vi "HandleTabTEST.vi"(8 "error in (no error)":errorcluster, 11 "S4GUI in":refnum<class "S4GUI.lvclass">) -> (0 "error out":errorcluster, 3 "S4GUI out":refnum<class "S4GUI.lvclass">)   [LabVIEW 2018, in "S4GUI.lvclass"]
uses:
  S4GUI.lvclass
  S4GUI.lvclass/S4GUI.ctl
  Instrument/Instrument.lvclass/Instrument.ctl
  Device/Optics/Optics.lvclass/Optics.ctl
  Device/Optics/Opt_Selector/Opt_Selector.lvclass
  C:/Users/devstaff/sparc4/s4gui/Versao ZeroMQ REQ-REP/SPARC4_GUI -v1.0.9 - novo comportamento aba TEST/Device/Optics/Optics.lvclass
  Acquisition/Acquisition.lvclass
  Instrument/Instrument.lvclass
  Channel/Channel.lvclass
  Interface/Interface.lvclass
  Device/Optics/Optics.lvclass
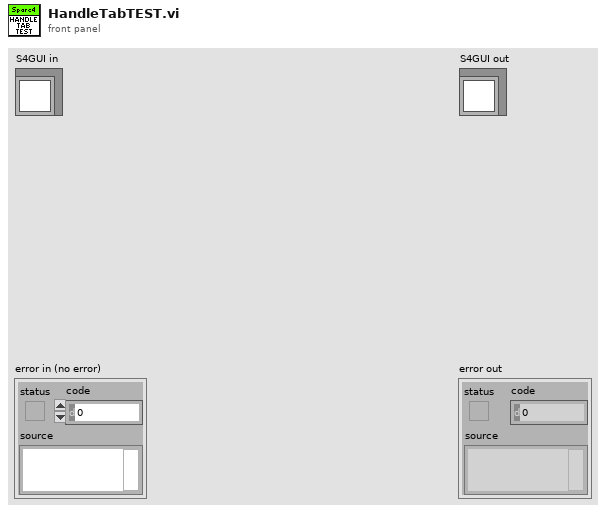
[diagram p1: front panel]
types:
  T1 = enum32{"OBJECT", "TEST", "DFLAT", "SFLAT", "DARK", "ZERO", "FOCUS"}
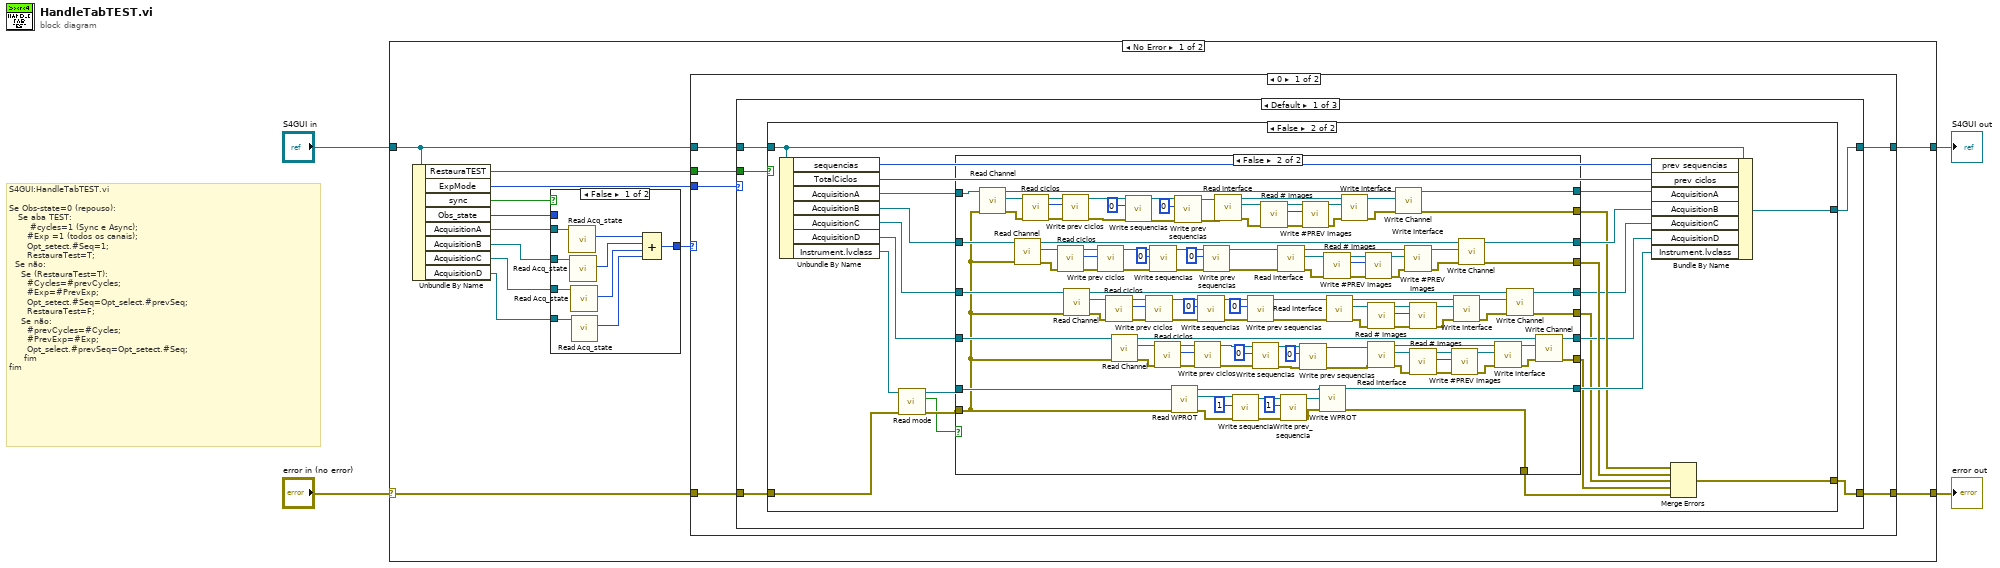
[diagram p0: block diagram]
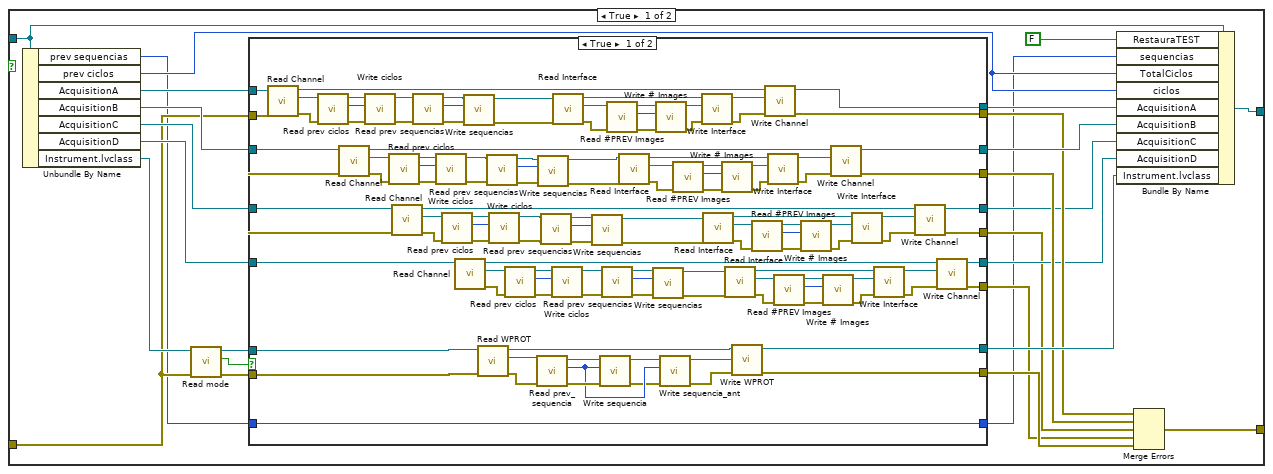
[diagram p3: hidden frame]
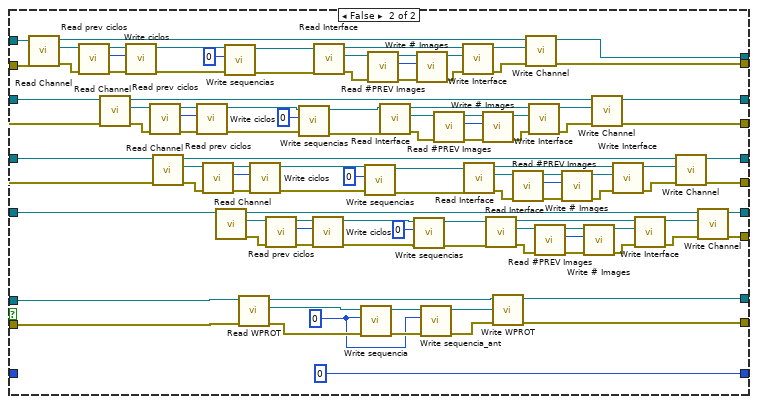
[diagram p4: hidden frame]
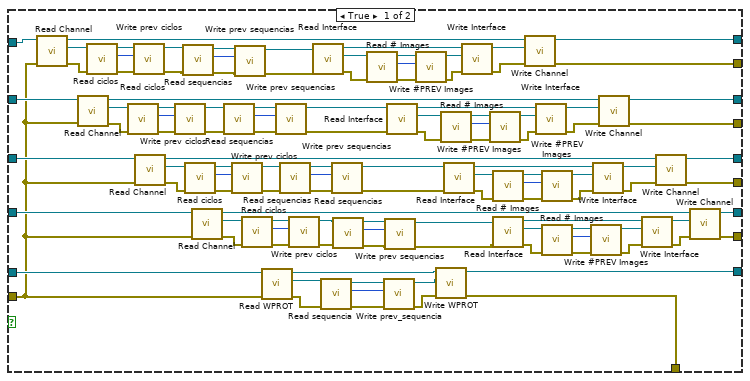
[diagram p5: hidden frame]
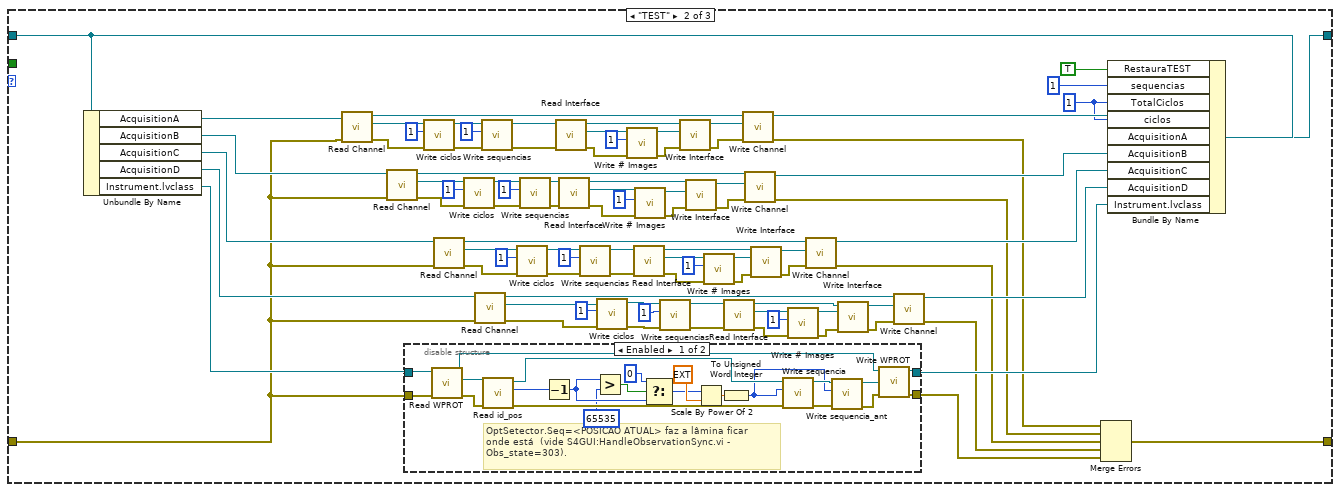
[diagram p6: hidden frame]
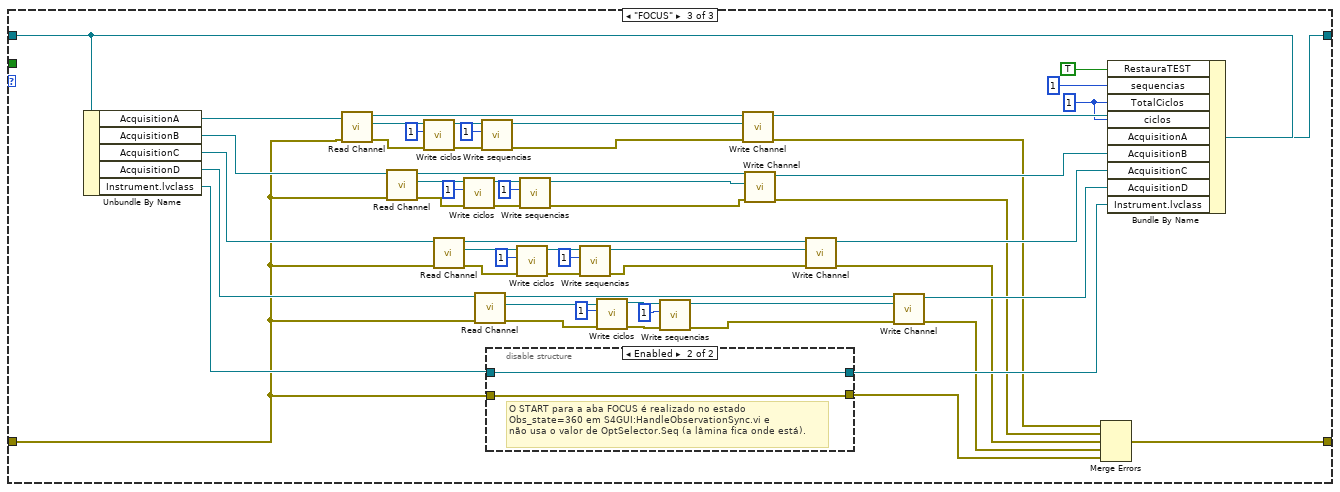
[diagram p8: hidden frame]
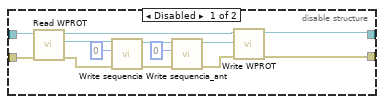
[diagram p9: hidden frame]
diagram:
  # "S4GUI:HandleTabTEST.vi\n\nSe Obs-state=0 (repouso):\n   Se aba TEST: \n       #cycles=1 (Sync e Async);\n      #Exp =1 (todos os canais);\n      Opt_setect.#Seq=1;\n      RestauraTest=T;\n  Se não:\n    Se (RestauraTest=T):\n      #Cycles=#prevCycles;\n      #Exp=#PrevExp;\n      Opt_setect.#Seq=Opt_select.#prevSeq;\n      RestauraTest=F;\n    Se não:\n      #prevCycles=#Cycles;\n      #PrevExp=#Exp;\n      Opt_select.#prevSeq=Opt_setect.#Seq;\n     fim\nfim"
  n1 = case shown="No Error" "error in (no error)" {
    selector: "error in (no error)" -> [w17 w746]
    tunnel: [w14 w746] -> w3
    tunnel: [w15 w745] -> w1
    tunnel: "S4GUI in" -> [w16 w745]
    frame No Error {
      n2 = Unbundle By Name(w16) -> ("RestauraTEST"=w5:bool, "ExpMode"=w7:T1, "sync"=w6:bool, "Obs_state"=w13:u32, "AcquisitionA"=w12:refnum<class "Acquisition.lvclass">, "AcquisitionB"=w11:refnum<class "Acquisition.lvclass">, "AcquisitionC"=w10:refnum<class "Acquisition.lvclass">, "AcquisitionD"=w9:refnum<class "Acquisition.lvclass">)
      n3 = case shown="False" w6 {
        tunnel: w13 -> [_ w27]
        tunnel: w12 -> [w26 _]
        tunnel: w11 -> [w24 _]
        tunnel: w10 -> [w23 _]
        tunnel: w9 -> [w22 _]
        tunnel: [w18 w27] -> w8
        frame False {
          n4 = call-dynamic "Read Acq_state.vi"("Acquisition in"=w26) -> ("Acq_state"=w25:u32)  [unwired: 8 in, 2 out]
          n5 = call-dynamic "Read Acq_state.vi"("Acquisition in"=w24) -> ("Acq_state"=w21:u32)  [unwired: 8 in, 2 out]
          n6 = call-dynamic "Read Acq_state.vi"("Acquisition in"=w23) -> ("Acq_state"=w20:u32)  [unwired: 8 in, 2 out]
          n7 = call-dynamic "Read Acq_state.vi"("Acquisition in"=w22) -> ("Acq_state"=w19:u32)  [unwired: 8 in, 2 out]
          n8 = Compound Arithmetic op=ADD(w25, w21, w20, w19) -> (w18:u32)
        }
        frame True {
        }
      }
      n9 = case shown="0" w8 {
        tunnel: w17 -> [w30 w743]
        tunnel: [w31 w744] -> w15
        tunnel: w16 -> [w32 w744]
        tunnel: [w29 w743] -> w14
        tunnel: w7 -> [w33 _]
        tunnel: w5 -> [w28 _]
        frame 0 {
          n10 = case shown="Default" w33 {
            tunnel: w32 -> [w37 w604 w710]
            tunnel: [w34 w603 w709] -> w31
            tunnel: w30 -> [w36 w590 w700]
            tunnel: [w35 w584 w694] -> w29
            tunnel: w28 -> [w38 _ _]
            frame Default {
              n11 = case shown="False" w38 {
                tunnel: w37 -> [w55 w308]
                tunnel: w36 -> [w45 w298]
                tunnel: [w56 w309] -> w35
                tunnel: [w54 w307] -> w34
                frame True {
                  n12 = Unbundle By Name(w55) -> ("prev sequencias"=w40:u32, "prev ciclos"=w42:u32, "AcquisitionA"=w64:refnum<class "Acquisition.lvclass">, "AcquisitionB"=w61:refnum<class "Acquisition.lvclass">, "AcquisitionC"=w53:refnum<class "Acquisition.lvclass">, "AcquisitionD"=w52:refnum<class "Acquisition.lvclass">, "Instrument.lvclass"=w46:refnum<class "Instrument.lvclass">)
                  n13 = call-dynamic "Read mode.vi"("error in (no error)"=w45, "Instrument in"=w46) -> ("error out"=w43:errorcluster, "mode"=w41:bool, "Instrument out"=w44:refnum<class "Instrument.lvclass">)  [unwired: 7 in]
                  n14 = case shown="True" w41 {
                    tunnel: w64 -> [w184 w294]
                    tunnel: [w178 w288] -> w63
                    tunnel: [w177 w287] -> w62
                    tunnel: w61 -> [w152 w262]
                    tunnel: [w148 w258] -> w60
                    tunnel: [w147 w257] -> w59
                    tunnel: [w146 w256] -> w58
                    tunnel: [w145 w255] -> w57
                    tunnel: w53 -> [w135 w245]
                    tunnel: w52 -> [w111 w221]
                    tunnel: [w110 w220] -> w51
                    tunnel: [w109 w219] -> w50
                    tunnel: [w108 w218] -> w49
                    tunnel: [w107 w217] -> w48
                    tunnel: w45 -> [w78 w208]
                    tunnel: w44 -> [w77 w207]
                    tunnel: w43 -> [w76 w206]
                    tunnel: w40 -> [w65 _]
                    tunnel: [w65 u32 0 ("prev sequencias")] -> w39
                    frame True {
                      n15 = call-dynamic "Read Channel.vi"("error in (no error)"=w78, "Acquisition in"=w184) -> ("error out"=w172:errorcluster, "Channel.lvclass"=w175:refnum<class "Channel.lvclass">, "Acquisition out"=w183:refnum<class "Acquisition.lvclass">)  [unwired: 7 in]
                      n16 = call-dynamic "Read prev ciclos.vi"("error in (no error)"=w172, "Channel in"=w175) -> ("error out"=w171:errorcluster, "prev ciclos"=w173:u32, "Channel out"=w174:refnum<class "Channel.lvclass">)  [unwired: 7 in]
                      n17 = call-dynamic "Read Channel.vi"("error in (no error)"=w78, "Acquisition in"=w152) -> ("error out"=w157:errorcluster, "Channel.lvclass"=w160:refnum<class "Channel.lvclass">, "Acquisition out"=w165:refnum<class "Acquisition.lvclass">)  [unwired: 7 in]
                      n18 = call-dynamic "Write ciclos.vi"("error in (no error)"=w171, "ciclos"=w173, "Channel in"=w174) -> ("error out"=w102:errorcluster, "Channel out"=w106:refnum<class "Channel.lvclass">)  [unwired: 7 in]
                      n19 = call-dynamic "Read prev ciclos.vi"("error in (no error)"=w157, "Channel in"=w160) -> ("error out"=w156:errorcluster, "prev ciclos"=w158:u32, "Channel out"=w159:refnum<class "Channel.lvclass">)  [unwired: 7 in]
                      n20 = call-dynamic "Read Channel.vi"("error in (no error)"=w78, "Acquisition in"=w135) -> ("error out"=w137:errorcluster, "Channel.lvclass"=w140:refnum<class "Channel.lvclass">, "Acquisition out"=w144:refnum<class "Acquisition.lvclass">)  [unwired: 7 in]
                      n21 = call-dynamic "Read prev sequencias.vi"("error in (no error)"=w102, "Channel in"=w106) -> ("error out"=w101:errorcluster, "prev sequencias"=w104:u32, "Channel out"=w105:refnum<class "Channel.lvclass">)  [unwired: 7 in]
                      n22 = call-dynamic "Write ciclos.vi"("error in (no error)"=w156, "ciclos"=w158, "Channel in"=w159) -> ("error out"=w90:errorcluster, "Channel out"=w93:refnum<class "Channel.lvclass">)  [unwired: 7 in]
                      n23 = call-dynamic "Read prev ciclos.vi"("error in (no error)"=w137, "Channel in"=w140) -> ("error out"=w136:errorcluster, "prev ciclos"=w138:u32, "Channel out"=w139:refnum<class "Channel.lvclass">)  [unwired: 7 in]
                      n24 = call-dynamic "Read Channel.vi"("Acquisition in"=w111) -> ("error out"=w120:errorcluster, "Channel.lvclass"=w123:refnum<class "Channel.lvclass">, "Acquisition out"=w127:refnum<class "Acquisition.lvclass">)  [unwired: 8 in]
                      n25 = call-dynamic "Write sequencias.vi"("error in (no error)"=w101, "sequencias"=w104, "Channel in"=w105) -> ("error out"=w100:errorcluster, "Channel out"=w103:refnum<class "Channel.lvclass">)  [unwired: 7 in]
                      n26 = call "Read WPROT.vi"("error in (no error)"=w76, "Instrument in"=w77) -> ("error out"=w72:errorcluster, "Opt_Selector.lvclass"=w74:refnum<class "Opt_Selector.lvclass">, "Instrument out"=w75:refnum<class "Instrument.lvclass">)  [unwired: 7 in]
                      n27 = call-dynamic "Read prev sequencias.vi"("error in (no error)"=w90, "Channel in"=w93) -> ("error out"=w98:errorcluster, "prev sequencias"=w99:u32, "Channel out"=w92:refnum<class "Channel.lvclass">)  [unwired: 7 in]
                      n28 = call-dynamic "Write ciclos.vi"("error in (no error)"=w136, "ciclos"=w138, "Channel in"=w139) -> ("error out"=w87:errorcluster, "Channel out"=w88:refnum<class "Channel.lvclass">)  [unwired: 7 in]
                      n29 = call-dynamic "Read prev ciclos.vi"("error in (no error)"=w120, "Channel in"=w123) -> ("error out"=w119:errorcluster, "prev ciclos"=w121:u32, "Channel out"=w122:refnum<class "Channel.lvclass">)  [unwired: 7 in]
                      n30 = call-dynamic "Read prev_sequencia.vi"("error in (no error)"=w72, "Opt_Selector in"=w74) -> ("error out"=w71:errorcluster, "prev_sequencia"=w70:u16, "Opt_Selector out"=w73:refnum<class "Opt_Selector.lvclass">)  [unwired: 7 in]
                      n31 = call-dynamic "Write sequencias.vi"("error in (no error)"=w98, "sequencias"=w99, "Channel in"=w92) -> ("error out"=w89:errorcluster, "Channel out"=w91:refnum<class "Channel.lvclass">)  [unwired: 7 in]
                      n32 = call-dynamic "Read prev sequencias.vi"("error in (no error)"=w87, "Channel in"=w88) -> ("error out"=w96:errorcluster, "prev sequencias"=w97:u32, "Channel out"=w86:refnum<class "Channel.lvclass">)  [unwired: 7 in]
                      n33 = call-dynamic "Write ciclos.vi"("error in (no error)"=w119, "ciclos"=w121, "Channel in"=w122) -> ("error out"=w81:errorcluster, "Channel out"=w83:refnum<class "Channel.lvclass">)  [unwired: 7 in]
                      n34 = call-dynamic "Read Interface.vi"("error in (no error)"=w100, "Channel in"=w103) -> ("error out"=w167:errorcluster, "Interface.lvclass"=w170:refnum<class "Interface.lvclass">, "Channel out"=w182:refnum<class "Channel.lvclass">)  [unwired: 7 in]
                      n35 = call-dynamic "Write sequencias.vi"("error in (no error)"=w96, "sequencias"=w97, "Channel in"=w86) -> ("error out"=w84:errorcluster, "Channel out"=w85:refnum<class "Channel.lvclass">)  [unwired: 7 in]
                      n36 = call-dynamic "Write sequencia.vi"("error in (no error)"=w71, "sequencia"=w70, "Opt_Selector in"=w73) -> ("error out"=w68:errorcluster, "Opt_Selector out"=w69:refnum<class "Opt_Selector.lvclass">)  [unwired: 7 in]
                      n37 = call-dynamic "Read prev sequencias.vi"("error in (no error)"=w81, "Channel in"=w83) -> ("error out"=w94:errorcluster, "prev sequencias"=w95:u32, "Channel out"=w82:refnum<class "Channel.lvclass">)  [unwired: 7 in]
                      n38 = call-dynamic "Read #PREV Images.vi"("error in (no error)"=w167, "Interface in"=w170) -> ("error out"=w166:errorcluster, "#PREV FRAMES"=w168:u32, "Interface out"=w169:refnum<class "Interface.lvclass">)  [unwired: 7 in]
                      n39 = call-dynamic "Read Interface.vi"("error in (no error)"=w89, "Channel in"=w91) -> ("error out"=w151:errorcluster, "Interface.lvclass"=w155:refnum<class "Interface.lvclass">, "Channel out"=w164:refnum<class "Channel.lvclass">)  [unwired: 7 in]
                      n40 = call-dynamic "Write sequencias.vi"("error in (no error)"=w94, "sequencias"=w95, "Channel in"=w82) -> ("error out"=w80:errorcluster, "Channel out"=w79:refnum<class "Channel.lvclass">)  [unwired: 7 in]
                      n41 = call-dynamic "Write # Images.vi"("error in (no error)"=w166, "# Images"=w168, "Interface in"=w169) -> ("error out"=w180:errorcluster, "Interface out"=w176:refnum<class "Interface.lvclass">)  [unwired: 7 in]
                      n42 = call-dynamic "Write sequencia_ant.vi"("error in (no error)"=w68, "sequencia_ant"=w70, "Opt_Selector in"=w69) -> ("error out"=w67:errorcluster, "Opt_Selector out"=w66:refnum<class "Opt_Selector.lvclass">)  [unwired: 7 in]
                      n43 = call-dynamic "Read #PREV Images.vi"("error in (no error)"=w151, "Interface in"=w155) -> ("error out"=w150:errorcluster, "#PREV FRAMES"=w153:u32, "Interface out"=w154:refnum<class "Interface.lvclass">)  [unwired: 7 in]
                      n44 = call-dynamic "Write Interface.vi"("error in (no error)"=w180, "Interface.lvclass"=w176, "Channel in"=w182) -> ("error out"=w179:errorcluster, "Channel out"=w181:refnum<class "Channel.lvclass">)  [unwired: 7 in]
                      n45 = call-dynamic "Read Interface.vi"("error in (no error)"=w84, "Channel in"=w85) -> ("error out"=w130:errorcluster, "Interface.lvclass"=w133:refnum<class "Interface.lvclass">, "Channel out"=w143:refnum<class "Channel.lvclass">)  [unwired: 7 in]
                      n46 = call-dynamic "Write # Images.vi"("error in (no error)"=w150, "# Images"=w153, "Interface in"=w154) -> ("error out"=w149:errorcluster, "Interface out"=w161:refnum<class "Interface.lvclass">)  [unwired: 7 in]
                      n47 = call-dynamic "Read Interface.vi"("error in (no error)"=w80, "Channel in"=w79) -> ("error out"=w114:errorcluster, "Interface.lvclass"=w117:refnum<class "Interface.lvclass">, "Channel out"=w126:refnum<class "Channel.lvclass">)  [unwired: 7 in]
                      n48 = call "Write WPROT.vi"("error in (no error)"=w67, "Opt_Selector.lvclass"=w66, "Instrument in"=w75) -> ("error out"=w145:errorcluster, "Instrument out"=w177:refnum<class "Instrument.lvclass">)  [unwired: 7 in]
                      n49 = call-dynamic "Read #PREV Images.vi"("error in (no error)"=w130, "Interface in"=w133) -> ("error out"=w129:errorcluster, "#PREV FRAMES"=w134:u32, "Interface out"=w132:refnum<class "Interface.lvclass">)  [unwired: 7 in]
                      n50 = call-dynamic "Write Channel.vi"("error in (no error)"=w179, "Channel.lvclass"=w181, "Acquisition in"=w183) -> ("error out"=w147:errorcluster, "Acquisition out"=w178:refnum<class "Acquisition.lvclass">)  [unwired: 7 in]
                      n51 = call-dynamic "Write Interface.vi"("error in (no error)"=w149, "Interface.lvclass"=w161, "Channel in"=w164) -> ("error out"=w162:errorcluster, "Channel out"=w163:refnum<class "Channel.lvclass">)  [unwired: 7 in]
                      n52 = call-dynamic "Read #PREV Images.vi"("error in (no error)"=w114, "Interface in"=w117) -> ("error out"=w113:errorcluster, "#PREV FRAMES"=w118:u32, "Interface out"=w116:refnum<class "Interface.lvclass">)  [unwired: 7 in]
                      n53 = call-dynamic "Write # Images.vi"("error in (no error)"=w129, "# Images"=w134, "Interface in"=w132) -> ("error out"=w128:errorcluster, "Interface out"=w131:refnum<class "Interface.lvclass">)  [unwired: 7 in]
                      n54 = call-dynamic "Write # Images.vi"("error in (no error)"=w113, "# Images"=w118, "Interface in"=w116) -> ("error out"=w112:errorcluster, "Interface out"=w115:refnum<class "Interface.lvclass">)  [unwired: 7 in]
                      n55 = call-dynamic "Write Channel.vi"("error in (no error)"=w162, "Channel.lvclass"=w163, "Acquisition in"=w165) -> ("error out"=w146:errorcluster, "Acquisition out"=w148:refnum<class "Acquisition.lvclass">)  [unwired: 7 in]
                      n56 = call-dynamic "Write Interface.vi"("error in (no error)"=w128, "Interface.lvclass"=w131, "Channel in"=w143) -> ("error out"=w141:errorcluster, "Channel out"=w142:refnum<class "Channel.lvclass">)  [unwired: 7 in]
                      n57 = call-dynamic "Write Interface.vi"("error in (no error)"=w112, "Interface.lvclass"=w115, "Channel in"=w126) -> ("error out"=w124:errorcluster, "Channel out"=w125:refnum<class "Channel.lvclass">)  [unwired: 7 in]
                      n58 = call-dynamic "Write Channel.vi"("error in (no error)"=w141, "Channel.lvclass"=w142, "Acquisition in"=w144) -> ("error out"=w108:errorcluster, "Acquisition out"=w109:refnum<class "Acquisition.lvclass">)  [unwired: 7 in]
                      n59 = call-dynamic "Write Channel.vi"("error in (no error)"=w124, "Channel.lvclass"=w125, "Acquisition in"=w127) -> ("error out"=w107:errorcluster, "Acquisition out"=w110:refnum<class "Acquisition.lvclass">)  [unwired: 7 in]
                    }
                    frame False {
                      w186 = u32 0 ("sequencias")
                      n60 = call-dynamic "Read Channel.vi"("error in (no error)"=w208, "Acquisition in"=w294) -> ("error out"=w282:errorcluster, "Channel.lvclass"=w285:refnum<class "Channel.lvclass">, "Acquisition out"=w293:refnum<class "Acquisition.lvclass">)  [unwired: 7 in]
                      n61 = call-dynamic "Read prev ciclos.vi"("error in (no error)"=w282, "Channel in"=w285) -> ("error out"=w281:errorcluster, "prev ciclos"=w283:u32, "Channel out"=w284:refnum<class "Channel.lvclass">)  [unwired: 7 in]
                      n62 = call-dynamic "Read Channel.vi"("error in (no error)"=w208, "Acquisition in"=w262) -> ("error out"=w267:errorcluster, "Channel.lvclass"=w270:refnum<class "Channel.lvclass">, "Acquisition out"=w275:refnum<class "Acquisition.lvclass">)  [unwired: 7 in]
                      n63 = call-dynamic "Write ciclos.vi"("error in (no error)"=w281, "ciclos"=w283, "Channel in"=w284) -> ("error out"=w199:errorcluster, "Channel out"=w200:refnum<class "Channel.lvclass">)  [unwired: 7 in]
                      n64 = call-dynamic "Read prev ciclos.vi"("error in (no error)"=w267, "Channel in"=w270) -> ("error out"=w266:errorcluster, "prev ciclos"=w268:u32, "Channel out"=w269:refnum<class "Channel.lvclass">)  [unwired: 7 in]
                      n65 = call-dynamic "Read Channel.vi"("error in (no error)"=w208, "Acquisition in"=w245) -> ("error out"=w247:errorcluster, "Channel.lvclass"=w250:refnum<class "Channel.lvclass">, "Acquisition out"=w254:refnum<class "Acquisition.lvclass">)  [unwired: 7 in]
                      n66 = call-dynamic "Write ciclos.vi"("error in (no error)"=w266, "ciclos"=w268, "Channel in"=w269) -> ("error out"=w196:errorcluster, "Channel out"=w197:refnum<class "Channel.lvclass">)  [unwired: 7 in]
                      n67 = call-dynamic "Read prev ciclos.vi"("error in (no error)"=w247, "Channel in"=w250) -> ("error out"=w246:errorcluster, "prev ciclos"=w248:u32, "Channel out"=w249:refnum<class "Channel.lvclass">)  [unwired: 7 in]
                      n68 = call-dynamic "Read Channel.vi"("Acquisition in"=w221) -> ("error out"=w230:errorcluster, "Channel.lvclass"=w233:refnum<class "Channel.lvclass">, "Acquisition out"=w237:refnum<class "Acquisition.lvclass">)  [unwired: 8 in]
                      n69 = call-dynamic "Write sequencias.vi"("error in (no error)"=w199, "sequencias"=u32 0, "Channel in"=w200) -> ("error out"=w215:errorcluster, "Channel out"=w216:refnum<class "Channel.lvclass">)  [unwired: 7 in]
                      n70 = call "Read WPROT.vi"("error in (no error)"=w206, "Instrument in"=w207) -> ("error out"=w187:errorcluster, "Opt_Selector.lvclass"=w188:refnum<class "Opt_Selector.lvclass">, "Instrument out"=w205:refnum<class "Instrument.lvclass">)  [unwired: 7 in]
                      n71 = call-dynamic "Write ciclos.vi"("error in (no error)"=w246, "ciclos"=w248, "Channel in"=w249) -> ("error out"=w193:errorcluster, "Channel out"=w194:refnum<class "Channel.lvclass">)  [unwired: 7 in]
                      n72 = call-dynamic "Read prev ciclos.vi"("error in (no error)"=w230, "Channel in"=w233) -> ("error out"=w229:errorcluster, "prev ciclos"=w231:u32, "Channel out"=w232:refnum<class "Channel.lvclass">)  [unwired: 7 in]
                      n73 = call-dynamic "Write sequencias.vi"("error in (no error)"=w196, "sequencias"=u32 0, "Channel in"=w197) -> ("error out"=w213:errorcluster, "Channel out"=w214:refnum<class "Channel.lvclass">)  [unwired: 7 in]
                      n74 = call-dynamic "Write ciclos.vi"("error in (no error)"=w229, "ciclos"=w231, "Channel in"=w232) -> ("error out"=w190:errorcluster, "Channel out"=w191:refnum<class "Channel.lvclass">)  [unwired: 7 in]
                      n75 = call-dynamic "Read Interface.vi"("error in (no error)"=w215, "Channel in"=w216) -> ("error out"=w277:errorcluster, "Interface.lvclass"=w280:refnum<class "Interface.lvclass">, "Channel out"=w292:refnum<class "Channel.lvclass">)  [unwired: 7 in]
                      n76 = call-dynamic "Write sequencia.vi"("error in (no error)"=w187, "sequencia"=w186, "Opt_Selector in"=w188) -> ("error out"=w203:errorcluster, "Opt_Selector out"=w204:refnum<class "Opt_Selector.lvclass">)  [unwired: 7 in]
                      n77 = call-dynamic "Write sequencias.vi"("error in (no error)"=w193, "sequencias"=u32 0, "Channel in"=w194) -> ("error out"=w211:errorcluster, "Channel out"=w212:refnum<class "Channel.lvclass">)  [unwired: 7 in]
                      n78 = call-dynamic "Read #PREV Images.vi"("error in (no error)"=w277, "Interface in"=w280) -> ("error out"=w276:errorcluster, "#PREV FRAMES"=w278:u32, "Interface out"=w279:refnum<class "Interface.lvclass">)  [unwired: 7 in]
                      n79 = call-dynamic "Read Interface.vi"("error in (no error)"=w213, "Channel in"=w214) -> ("error out"=w261:errorcluster, "Interface.lvclass"=w265:refnum<class "Interface.lvclass">, "Channel out"=w274:refnum<class "Channel.lvclass">)  [unwired: 7 in]
                      n80 = call-dynamic "Write sequencias.vi"("error in (no error)"=w190, "sequencias"=u32 0, "Channel in"=w191) -> ("error out"=w210:errorcluster, "Channel out"=w209:refnum<class "Channel.lvclass">)  [unwired: 7 in]
                      n81 = call-dynamic "Write # Images.vi"("error in (no error)"=w276, "# Images"=w278, "Interface in"=w279) -> ("error out"=w290:errorcluster, "Interface out"=w286:refnum<class "Interface.lvclass">)  [unwired: 7 in]
                      n82 = call-dynamic "Write sequencia_ant.vi"("error in (no error)"=w203, "sequencia_ant"=w186, "Opt_Selector in"=w204) -> ("error out"=w202:errorcluster, "Opt_Selector out"=w201:refnum<class "Opt_Selector.lvclass">)  [unwired: 7 in]
                      n83 = call-dynamic "Read #PREV Images.vi"("error in (no error)"=w261, "Interface in"=w265) -> ("error out"=w260:errorcluster, "#PREV FRAMES"=w263:u32, "Interface out"=w264:refnum<class "Interface.lvclass">)  [unwired: 7 in]
                      n84 = call-dynamic "Write Interface.vi"("error in (no error)"=w290, "Interface.lvclass"=w286, "Channel in"=w292) -> ("error out"=w289:errorcluster, "Channel out"=w291:refnum<class "Channel.lvclass">)  [unwired: 7 in]
                      n85 = call-dynamic "Read Interface.vi"("error in (no error)"=w211, "Channel in"=w212) -> ("error out"=w240:errorcluster, "Interface.lvclass"=w243:refnum<class "Interface.lvclass">, "Channel out"=w253:refnum<class "Channel.lvclass">)  [unwired: 7 in]
                      n86 = call-dynamic "Write # Images.vi"("error in (no error)"=w260, "# Images"=w263, "Interface in"=w264) -> ("error out"=w259:errorcluster, "Interface out"=w271:refnum<class "Interface.lvclass">)  [unwired: 7 in]
                      n87 = call-dynamic "Read Interface.vi"("error in (no error)"=w210, "Channel in"=w209) -> ("error out"=w224:errorcluster, "Interface.lvclass"=w227:refnum<class "Interface.lvclass">, "Channel out"=w236:refnum<class "Channel.lvclass">)  [unwired: 7 in]
                      n88 = call "Write WPROT.vi"("error in (no error)"=w202, "Opt_Selector.lvclass"=w201, "Instrument in"=w205) -> ("error out"=w255:errorcluster, "Instrument out"=w287:refnum<class "Instrument.lvclass">)  [unwired: 7 in]
                      n89 = call-dynamic "Read #PREV Images.vi"("error in (no error)"=w240, "Interface in"=w243) -> ("error out"=w239:errorcluster, "#PREV FRAMES"=w244:u32, "Interface out"=w242:refnum<class "Interface.lvclass">)  [unwired: 7 in]
                      n90 = call-dynamic "Write Channel.vi"("error in (no error)"=w289, "Channel.lvclass"=w291, "Acquisition in"=w293) -> ("error out"=w257:errorcluster, "Acquisition out"=w288:refnum<class "Acquisition.lvclass">)  [unwired: 7 in]
                      n91 = call-dynamic "Write Interface.vi"("error in (no error)"=w259, "Interface.lvclass"=w271, "Channel in"=w274) -> ("error out"=w272:errorcluster, "Channel out"=w273:refnum<class "Channel.lvclass">)  [unwired: 7 in]
                      n92 = call-dynamic "Read #PREV Images.vi"("error in (no error)"=w224, "Interface in"=w227) -> ("error out"=w223:errorcluster, "#PREV FRAMES"=w228:u32, "Interface out"=w226:refnum<class "Interface.lvclass">)  [unwired: 7 in]
                      n93 = call-dynamic "Write # Images.vi"("error in (no error)"=w239, "# Images"=w244, "Interface in"=w242) -> ("error out"=w238:errorcluster, "Interface out"=w241:refnum<class "Interface.lvclass">)  [unwired: 7 in]
                      n94 = call-dynamic "Write # Images.vi"("error in (no error)"=w223, "# Images"=w228, "Interface in"=w226) -> ("error out"=w222:errorcluster, "Interface out"=w225:refnum<class "Interface.lvclass">)  [unwired: 7 in]
                      n95 = call-dynamic "Write Channel.vi"("error in (no error)"=w272, "Channel.lvclass"=w273, "Acquisition in"=w275) -> ("error out"=w256:errorcluster, "Acquisition out"=w258:refnum<class "Acquisition.lvclass">)  [unwired: 7 in]
                      n96 = call-dynamic "Write Interface.vi"("error in (no error)"=w238, "Interface.lvclass"=w241, "Channel in"=w253) -> ("error out"=w251:errorcluster, "Channel out"=w252:refnum<class "Channel.lvclass">)  [unwired: 7 in]
                      n97 = call-dynamic "Write Interface.vi"("error in (no error)"=w222, "Interface.lvclass"=w225, "Channel in"=w236) -> ("error out"=w234:errorcluster, "Channel out"=w235:refnum<class "Channel.lvclass">)  [unwired: 7 in]
                      n98 = call-dynamic "Write Channel.vi"("error in (no error)"=w251, "Channel.lvclass"=w252, "Acquisition in"=w254) -> ("error out"=w218:errorcluster, "Acquisition out"=w219:refnum<class "Acquisition.lvclass">)  [unwired: 7 in]
                      n99 = call-dynamic "Write Channel.vi"("error in (no error)"=w234, "Channel.lvclass"=w235, "Acquisition in"=w237) -> ("error out"=w217:errorcluster, "Acquisition out"=w220:refnum<class "Acquisition.lvclass">)  [unwired: 7 in]
                    }
                  }
                  n100 = Bundle By Name(cluster=w55, "RestauraTEST"=FALSE, "sequencias"=w39, "TotalCiclos"=w42, "ciclos"=w42, "AcquisitionA"=w63, "AcquisitionB"=w60, "AcquisitionC"=w50, "AcquisitionD"=w51, "Instrument.lvclass"=w62) -> (w54:refnum<class "S4GUI.lvclass">)
                  n101 = Merge Errors(w59, w58, w49, w48, w57) -> (w56:errorcluster)
                }
                frame False {
                  n102 = Unbundle By Name(w308) -> ("sequencias"=w300:u32, "TotalCiclos"=w315:u32, "AcquisitionA"=w318:refnum<class "Acquisition.lvclass">, "AcquisitionB"=w314:refnum<class "Acquisition.lvclass">, "AcquisitionC"=w306:refnum<class "Acquisition.lvclass">, "AcquisitionD"=w305:refnum<class "Acquisition.lvclass">, "Instrument.lvclass"=w299:refnum<class "Instrument.lvclass">)
                  n103 = call-dynamic "Read mode.vi"("error in (no error)"=w298, "Instrument in"=w299) -> ("error out"=w297:errorcluster, "mode"=w295:bool, "Instrument out"=w296:refnum<class "Instrument.lvclass">)  [unwired: 7 in]
                  n104 = case shown="False" w295 {
                    tunnel: w318 -> [w434 w555]
                    tunnel: w296 -> [w433 w554]
                    tunnel: [w425 w546] -> w317
                    tunnel: [w424 w545] -> w316
                    tunnel: w314 -> [w398 w519]
                    tunnel: [w394 w515] -> w313
                    tunnel: [w393 w514] -> w312
                    tunnel: [w392 w513] -> w311
                    tunnel: [w391 w512] -> w310
                    tunnel: w306 -> [w381 w502]
                    tunnel: w297 -> [w319 w445]
                    tunnel: w305 -> [w357 w478]
                    tunnel: [w356 w477] -> w304
                    tunnel: [w355 w476] -> w303
                    tunnel: [w354 w475] -> w302
                    tunnel: [w353 w474] -> w301
                    frame True {
                      n105 = call-dynamic "Read Channel.vi"("error in (no error)"=w319, "Acquisition in"=w434) -> ("error out"=w418:errorcluster, "Channel.lvclass"=w421:refnum<class "Channel.lvclass">, "Acquisition out"=w432:refnum<class "Acquisition.lvclass">)  [unwired: 7 in]
                      n106 = call-dynamic "Read Channel.vi"("error in (no error)"=w319, "Acquisition in"=w398) -> ("error out"=w403:errorcluster, "Channel.lvclass"=w406:refnum<class "Channel.lvclass">, "Acquisition out"=w411:refnum<class "Acquisition.lvclass">)  [unwired: 7 in]
                      n107 = call-dynamic "Read ciclos.vi"("error in (no error)"=w418, "Channel in"=w421) -> ("error out"=w417:errorcluster, "ciclos"=w419:u32, "Channel out"=w420:refnum<class "Channel.lvclass">)  [unwired: 7 in]
                      n108 = call-dynamic "Read ciclos.vi"("error in (no error)"=w403, "Channel in"=w406) -> ("error out"=w402:errorcluster, "ciclos"=w404:u32, "Channel out"=w405:refnum<class "Channel.lvclass">)  [unwired: 7 in]
                      n109 = call-dynamic "Write prev ciclos.vi"("error in (no error)"=w417, "prev ciclos"=w419, "Channel in"=w420) -> ("error out"=w344:errorcluster, "Channel out"=w347:refnum<class "Channel.lvclass">)  [unwired: 7 in]
                      n110 = call-dynamic "Read Channel.vi"("error in (no error)"=w319, "Acquisition in"=w381) -> ("error out"=w383:errorcluster, "Channel.lvclass"=w386:refnum<class "Channel.lvclass">, "Acquisition out"=w390:refnum<class "Acquisition.lvclass">)  [unwired: 7 in]
                      n111 = call-dynamic "Write prev ciclos.vi"("error in (no error)"=w402, "prev ciclos"=w404, "Channel in"=w405) -> ("error out"=w333:errorcluster, "Channel out"=w334:refnum<class "Channel.lvclass">)  [unwired: 7 in]
                      n112 = call-dynamic "Read sequencias.vi"("error in (no error)"=w344, "Channel in"=w347) -> ("error out"=w343:errorcluster, "sequencias"=w345:u32, "Channel out"=w346:refnum<class "Channel.lvclass">)  [unwired: 7 in]
                      n113 = call-dynamic "Read ciclos.vi"("error in (no error)"=w383, "Channel in"=w386) -> ("error out"=w382:errorcluster, "ciclos"=w384:u32, "Channel out"=w385:refnum<class "Channel.lvclass">)  [unwired: 7 in]
                      n114 = call-dynamic "Read Channel.vi"("error in (no error)"=w319, "Acquisition in"=w357) -> ("error out"=w366:errorcluster, "Channel.lvclass"=w369:refnum<class "Channel.lvclass">, "Acquisition out"=w373:refnum<class "Acquisition.lvclass">)  [unwired: 7 in]
                      n115 = call-dynamic "Read sequencias.vi"("error in (no error)"=w333, "Channel in"=w334) -> ("error out"=w339:errorcluster, "sequencias"=w340:u32, "Channel out"=w332:refnum<class "Channel.lvclass">)  [unwired: 7 in]
                      n116 = call-dynamic "Write prev ciclos.vi"("error in (no error)"=w382, "prev ciclos"=w384, "Channel in"=w385) -> ("error out"=w328:errorcluster, "Channel out"=w329:refnum<class "Channel.lvclass">)  [unwired: 7 in]
                      n117 = call-dynamic "Write prev sequencias.vi"("error in (no error)"=w343, "prev sequencias"=w345, "Channel in"=w346) -> ("error out"=w342:errorcluster, "Channel out"=w341:refnum<class "Channel.lvclass">)  [unwired: 7 in]
                      n118 = call-dynamic "Read ciclos.vi"("error in (no error)"=w366, "Channel in"=w369) -> ("error out"=w365:errorcluster, "ciclos"=w367:u32, "Channel out"=w368:refnum<class "Channel.lvclass">)  [unwired: 7 in]
                      n119 = call "Read WPROT.vi"("error in (no error)"=w319, "Instrument in"=w433) -> ("error out"=w349:errorcluster, "Opt_Selector.lvclass"=w352:refnum<class "Opt_Selector.lvclass">, "Instrument out"=w427:refnum<class "Instrument.lvclass">)  [unwired: 7 in]
                      n120 = call-dynamic "Write prev sequencias.vi"("error in (no error)"=w339, "prev sequencias"=w340, "Channel in"=w332) -> ("error out"=w330:errorcluster, "Channel out"=w331:refnum<class "Channel.lvclass">)  [unwired: 7 in]
                      n121 = call-dynamic "Read sequencias.vi"("error in (no error)"=w328, "Channel in"=w329) -> ("error out"=w337:errorcluster, "sequencias"=w338:u32, "Channel out"=w327:refnum<class "Channel.lvclass">)  [unwired: 7 in]
                      n122 = call-dynamic "Write prev ciclos.vi"("error in (no error)"=w365, "prev ciclos"=w367, "Channel in"=w368) -> ("error out"=w323:errorcluster, "Channel out"=w324:refnum<class "Channel.lvclass">)  [unwired: 7 in]
                      n123 = call-dynamic "Read Interface.vi"("error in (no error)"=w342, "Channel in"=w341) -> ("error out"=w413:errorcluster, "Interface.lvclass"=w416:refnum<class "Interface.lvclass">, "Channel out"=w431:refnum<class "Channel.lvclass">)  [unwired: 7 in]
                      n124 = call-dynamic "Read sequencia.vi"("error in (no error)"=w349, "Opt_Selector in"=w352) -> ("error out"=w348:errorcluster, "sequencia"=w350:u16, "Opt_Selector out"=w351:refnum<class "Opt_Selector.lvclass">)  [unwired: 7 in]
                      n125 = call-dynamic "Write prev sequencias.vi"("error in (no error)"=w337, "prev sequencias"=w338, "Channel in"=w327) -> ("error out"=w325:errorcluster, "Channel out"=w326:refnum<class "Channel.lvclass">)  [unwired: 7 in]
                      n126 = call-dynamic "Read sequencias.vi"("error in (no error)"=w323, "Channel in"=w324) -> ("error out"=w335:errorcluster, "sequencias"=w336:u32, "Channel out"=w322:refnum<class "Channel.lvclass">)  [unwired: 7 in]
                      n127 = call-dynamic "Read # Images.vi"("error in (no error)"=w413, "Interface in"=w416) -> ("error out"=w412:errorcluster, "# Images"=w414:u32, "Interface out"=w415:refnum<class "Interface.lvclass">)  [unwired: 7 in]
                      n128 = call-dynamic "Write prev_sequencia.vi"("error in (no error)"=w348, "prev_sequencia"=w350, "Opt_Selector in"=w351) -> ("error out"=w423:errorcluster, "Opt_Selector out"=w426:refnum<class "Opt_Selector.lvclass">)  [unwired: 7 in]
                      n129 = call-dynamic "Write prev sequencias.vi"("error in (no error)"=w335, "prev sequencias"=w336, "Channel in"=w322) -> ("error out"=w320:errorcluster, "Channel out"=w321:refnum<class "Channel.lvclass">)  [unwired: 7 in]
                      n130 = call-dynamic "Read Interface.vi"("error in (no error)"=w330, "Channel in"=w331) -> ("error out"=w397:errorcluster, "Interface.lvclass"=w401:refnum<class "Interface.lvclass">, "Channel out"=w410:refnum<class "Channel.lvclass">)  [unwired: 7 in]
                      n131 = call-dynamic "Write #PREV Images.vi"("error in (no error)"=w412, "#PREV FRAMES"=w414, "Interface in"=w415) -> ("error out"=w429:errorcluster, "Interface out"=w422:refnum<class "Interface.lvclass">)  [unwired: 7 in]
                      n132 = call "Write WPROT.vi"("error in (no error)"=w423, "Opt_Selector.lvclass"=w426, "Instrument in"=w427) -> ("error out"=w391:errorcluster, "Instrument out"=w424:refnum<class "Instrument.lvclass">)  [unwired: 7 in]
                      n133 = call-dynamic "Read # Images.vi"("error in (no error)"=w397, "Interface in"=w401) -> ("error out"=w396:errorcluster, "# Images"=w399:u32, "Interface out"=w400:refnum<class "Interface.lvclass">)  [unwired: 7 in]
                      n134 = call-dynamic "Read Interface.vi"("error in (no error)"=w325, "Channel in"=w326) -> ("error out"=w376:errorcluster, "Interface.lvclass"=w379:refnum<class "Interface.lvclass">, "Channel out"=w389:refnum<class "Channel.lvclass">)  [unwired: 7 in]
                      n135 = call-dynamic "Write Interface.vi"("error in (no error)"=w429, "Interface.lvclass"=w422, "Channel in"=w431) -> ("error out"=w428:errorcluster, "Channel out"=w430:refnum<class "Channel.lvclass">)  [unwired: 7 in]
                      n136 = call-dynamic "Write #PREV Images.vi"("error in (no error)"=w396, "#PREV FRAMES"=w399, "Interface in"=w400) -> ("error out"=w395:errorcluster, "Interface out"=w407:refnum<class "Interface.lvclass">)  [unwired: 7 in]
                      n137 = call-dynamic "Read # Images.vi"("error in (no error)"=w376, "Interface in"=w379) -> ("error out"=w375:errorcluster, "# Images"=w380:u32, "Interface out"=w378:refnum<class "Interface.lvclass">)  [unwired: 7 in]
                      n138 = call-dynamic "Read Interface.vi"("error in (no error)"=w320, "Channel in"=w321) -> ("error out"=w360:errorcluster, "Interface.lvclass"=w363:refnum<class "Interface.lvclass">, "Channel out"=w372:refnum<class "Channel.lvclass">)  [unwired: 7 in]
                      n139 = call-dynamic "Write Channel.vi"("error in (no error)"=w428, "Channel.lvclass"=w430, "Acquisition in"=w432) -> ("error out"=w393:errorcluster, "Acquisition out"=w425:refnum<class "Acquisition.lvclass">)  [unwired: 7 in]
                      n140 = call-dynamic "Write Interface.vi"("error in (no error)"=w395, "Interface.lvclass"=w407, "Channel in"=w410) -> ("error out"=w408:errorcluster, "Channel out"=w409:refnum<class "Channel.lvclass">)  [unwired: 7 in]
                      n141 = call-dynamic "Write #PREV Images.vi"("error in (no error)"=w375, "#PREV FRAMES"=w380, "Interface in"=w378) -> ("error out"=w374:errorcluster, "Interface out"=w377:refnum<class "Interface.lvclass">)  [unwired: 7 in]
                      n142 = call-dynamic "Read # Images.vi"("error in (no error)"=w360, "Interface in"=w363) -> ("error out"=w359:errorcluster, "# Images"=w364:u32, "Interface out"=w362:refnum<class "Interface.lvclass">)  [unwired: 7 in]
                      n143 = call-dynamic "Write #PREV Images.vi"("error in (no error)"=w359, "#PREV FRAMES"=w364, "Interface in"=w362) -> ("error out"=w358:errorcluster, "Interface out"=w361:refnum<class "Interface.lvclass">)  [unwired: 7 in]
                      n144 = call-dynamic "Write Interface.vi"("error in (no error)"=w374, "Interface.lvclass"=w377, "Channel in"=w389) -> ("error out"=w387:errorcluster, "Channel out"=w388:refnum<class "Channel.lvclass">)  [unwired: 7 in]
                      n145 = call-dynamic "Write Channel.vi"("error in (no error)"=w408, "Channel.lvclass"=w409, "Acquisition in"=w411) -> ("error out"=w392:errorcluster, "Acquisition out"=w394:refnum<class "Acquisition.lvclass">)  [unwired: 7 in]
                      n146 = call-dynamic "Write Interface.vi"("error in (no error)"=w358, "Interface.lvclass"=w361, "Channel in"=w372) -> ("error out"=w370:errorcluster, "Channel out"=w371:refnum<class "Channel.lvclass">)  [unwired: 7 in]
                      n147 = call-dynamic "Write Channel.vi"("error in (no error)"=w387, "Channel.lvclass"=w388, "Acquisition in"=w390) -> ("error out"=w354:errorcluster, "Acquisition out"=w355:refnum<class "Acquisition.lvclass">)  [unwired: 7 in]
                      n148 = call-dynamic "Write Channel.vi"("error in (no error)"=w370, "Channel.lvclass"=w371, "Acquisition in"=w373) -> ("error out"=w353:errorcluster, "Acquisition out"=w356:refnum<class "Acquisition.lvclass">)  [unwired: 7 in]
                    }
                    frame False {
                      n149 = call-dynamic "Read Channel.vi"("error in (no error)"=w445, "Acquisition in"=w555) -> ("error out"=w539:errorcluster, "Channel.lvclass"=w542:refnum<class "Channel.lvclass">, "Acquisition out"=w553:refnum<class "Acquisition.lvclass">)  [unwired: 7 in]
                      n150 = call-dynamic "Read Channel.vi"("error in (no error)"=w445, "Acquisition in"=w519) -> ("error out"=w524:errorcluster, "Channel.lvclass"=w527:refnum<class "Channel.lvclass">, "Acquisition out"=w532:refnum<class "Acquisition.lvclass">)  [unwired: 7 in]
                      n151 = call-dynamic "Read ciclos.vi"("error in (no error)"=w539, "Channel in"=w542) -> ("error out"=w538:errorcluster, "ciclos"=w540:u32, "Channel out"=w541:refnum<class "Channel.lvclass">)  [unwired: 7 in]
                      n152 = call-dynamic "Read ciclos.vi"("error in (no error)"=w524, "Channel in"=w527) -> ("error out"=w523:errorcluster, "ciclos"=w525:u32, "Channel out"=w526:refnum<class "Channel.lvclass">)  [unwired: 7 in]
                      n153 = call-dynamic "Write prev ciclos.vi"("error in (no error)"=w538, "prev ciclos"=w540, "Channel in"=w541) -> ("error out"=w467:errorcluster, "Channel out"=w469:refnum<class "Channel.lvclass">)  [unwired: 7 in]
                      n154 = call-dynamic "Read Channel.vi"("error in (no error)"=w445, "Acquisition in"=w502) -> ("error out"=w504:errorcluster, "Channel.lvclass"=w507:refnum<class "Channel.lvclass">, "Acquisition out"=w511:refnum<class "Acquisition.lvclass">)  [unwired: 7 in]
                      n155 = call-dynamic "Write prev ciclos.vi"("error in (no error)"=w523, "prev ciclos"=w525, "Channel in"=w526) -> ("error out"=w459:errorcluster, "Channel out"=w460:refnum<class "Channel.lvclass">)  [unwired: 7 in]
                      n156 = call-dynamic "Read ciclos.vi"("error in (no error)"=w504, "Channel in"=w507) -> ("error out"=w503:errorcluster, "ciclos"=w505:u32, "Channel out"=w506:refnum<class "Channel.lvclass">)  [unwired: 7 in]
                      n157 = call-dynamic "Read Channel.vi"("error in (no error)"=w445, "Acquisition in"=w478) -> ("error out"=w487:errorcluster, "Channel.lvclass"=w490:refnum<class "Channel.lvclass">, "Acquisition out"=w494:refnum<class "Acquisition.lvclass">)  [unwired: 7 in]
                      n158 = call-dynamic "Write sequencias.vi"("error in (no error)"=w467, "sequencias"=u32 0, "Channel in"=w469) -> ("error out"=w466:errorcluster, "Channel out"=w468:refnum<class "Channel.lvclass">)  [unwired: 7 in]
                      n159 = call-dynamic "Write prev ciclos.vi"("error in (no error)"=w503, "prev ciclos"=w505, "Channel in"=w506) -> ("error out"=w454:errorcluster, "Channel out"=w455:refnum<class "Channel.lvclass">)  [unwired: 7 in]
                      n160 = call-dynamic "Write sequencias.vi"("error in (no error)"=w459, "sequencias"=u32 0, "Channel in"=w460) -> ("error out"=w463:errorcluster, "Channel out"=w458:refnum<class "Channel.lvclass">)  [unwired: 7 in]
                      n161 = call-dynamic "Read ciclos.vi"("error in (no error)"=w487, "Channel in"=w490) -> ("error out"=w486:errorcluster, "ciclos"=w488:u32, "Channel out"=w489:refnum<class "Channel.lvclass">)  [unwired: 7 in]
                      n162 = call "Read WPROT.vi"("error in (no error)"=w445, "Instrument in"=w554) -> ("error out"=w471:errorcluster, "Opt_Selector.lvclass"=w473:refnum<class "Opt_Selector.lvclass">, "Instrument out"=w548:refnum<class "Instrument.lvclass">)  [unwired: 7 in]
                      n163 = call-dynamic "Write prev sequencias.vi"("error in (no error)"=w466, "prev sequencias"=u32 0, "Channel in"=w468) -> ("error out"=w465:errorcluster, "Channel out"=w464:refnum<class "Channel.lvclass">)  [unwired: 7 in]
                      n164 = call-dynamic "Write prev ciclos.vi"("error in (no error)"=w486, "prev ciclos"=w488, "Channel in"=w489) -> ("error out"=w449:errorcluster, "Channel out"=w450:refnum<class "Channel.lvclass">)  [unwired: 7 in]
                      n165 = call-dynamic "Write sequencias.vi"("error in (no error)"=w454, "sequencias"=u32 0, "Channel in"=w455) -> ("error out"=w462:errorcluster, "Channel out"=w453:refnum<class "Channel.lvclass">)  [unwired: 7 in]
                      n166 = call-dynamic "Write prev sequencias.vi"("error in (no error)"=w463, "prev sequencias"=u32 0, "Channel in"=w458) -> ("error out"=w456:errorcluster, "Channel out"=w457:refnum<class "Channel.lvclass">)  [unwired: 7 in]
                      n167 = call-dynamic "Read Interface.vi"("error in (no error)"=w465, "Channel in"=w464) -> ("error out"=w534:errorcluster, "Interface.lvclass"=w537:refnum<class "Interface.lvclass">, "Channel out"=w552:refnum<class "Channel.lvclass">)  [unwired: 7 in]
                      n168 = call-dynamic "Write sequencia.vi"("error in (no error)"=w471, "sequencia"=u16 1, "Opt_Selector in"=w473) -> ("error out"=w470:errorcluster, "Opt_Selector out"=w472:refnum<class "Opt_Selector.lvclass">)  [unwired: 7 in]
                      n169 = call-dynamic "Write prev sequencias.vi"("error in (no error)"=w462, "prev sequencias"=u32 0, "Channel in"=w453) -> ("error out"=w451:errorcluster, "Channel out"=w452:refnum<class "Channel.lvclass">)  [unwired: 7 in]
                      n170 = call-dynamic "Write sequencias.vi"("error in (no error)"=w449, "sequencias"=u32 0, "Channel in"=w450) -> ("error out"=w461:errorcluster, "Channel out"=w448:refnum<class "Channel.lvclass">)  [unwired: 7 in]
                      n171 = call-dynamic "Read # Images.vi"("error in (no error)"=w534, "Interface in"=w537) -> ("error out"=w533:errorcluster, "# Images"=w535:u32, "Interface out"=w536:refnum<class "Interface.lvclass">)  [unwired: 7 in]
                      n172 = call-dynamic "Read Interface.vi"("error in (no error)"=w456, "Channel in"=w457) -> ("error out"=w518:errorcluster, "Interface.lvclass"=w522:refnum<class "Interface.lvclass">, "Channel out"=w531:refnum<class "Channel.lvclass">)  [unwired: 7 in]
                      n173 = call-dynamic "Write prev_sequencia.vi"("error in (no error)"=w470, "prev_sequencia"=u16 1, "Opt_Selector in"=w472) -> ("error out"=w544:errorcluster, "Opt_Selector out"=w547:refnum<class "Opt_Selector.lvclass">)  [unwired: 7 in]
                      n174 = call-dynamic "Write prev sequencias.vi"("error in (no error)"=w461, "prev sequencias"=u32 0, "Channel in"=w448) -> ("error out"=w446:errorcluster, "Channel out"=w447:refnum<class "Channel.lvclass">)  [unwired: 7 in]
                      n175 = call-dynamic "Write #PREV Images.vi"("error in (no error)"=w533, "#PREV FRAMES"=w535, "Interface in"=w536) -> ("error out"=w550:errorcluster, "Interface out"=w543:refnum<class "Interface.lvclass">)  [unwired: 7 in]
                      n176 = call "Write WPROT.vi"("error in (no error)"=w544, "Opt_Selector.lvclass"=w547, "Instrument in"=w548) -> ("error out"=w512:errorcluster, "Instrument out"=w545:refnum<class "Instrument.lvclass">)  [unwired: 7 in]
                      n177 = call-dynamic "Read # Images.vi"("error in (no error)"=w518, "Interface in"=w522) -> ("error out"=w517:errorcluster, "# Images"=w520:u32, "Interface out"=w521:refnum<class "Interface.lvclass">)  [unwired: 7 in]
                      n178 = call-dynamic "Read Interface.vi"("error in (no error)"=w451, "Channel in"=w452) -> ("error out"=w497:errorcluster, "Interface.lvclass"=w500:refnum<class "Interface.lvclass">, "Channel out"=w510:refnum<class "Channel.lvclass">)  [unwired: 7 in]
                      n179 = call-dynamic "Write Interface.vi"("error in (no error)"=w550, "Interface.lvclass"=w543, "Channel in"=w552) -> ("error out"=w549:errorcluster, "Channel out"=w551:refnum<class "Channel.lvclass">)  [unwired: 7 in]
                      n180 = call-dynamic "Write #PREV Images.vi"("error in (no error)"=w517, "#PREV FRAMES"=w520, "Interface in"=w521) -> ("error out"=w516:errorcluster, "Interface out"=w528:refnum<class "Interface.lvclass">)  [unwired: 7 in]
                      n181 = call-dynamic "Read # Images.vi"("error in (no error)"=w497, "Interface in"=w500) -> ("error out"=w496:errorcluster, "# Images"=w501:u32, "Interface out"=w499:refnum<class "Interface.lvclass">)  [unwired: 7 in]
                      n182 = call-dynamic "Read Interface.vi"("error in (no error)"=w446, "Channel in"=w447) -> ("error out"=w481:errorcluster, "Interface.lvclass"=w484:refnum<class "Interface.lvclass">, "Channel out"=w493:refnum<class "Channel.lvclass">)  [unwired: 7 in]
                      n183 = call-dynamic "Write Channel.vi"("error in (no error)"=w549, "Channel.lvclass"=w551, "Acquisition in"=w553) -> ("error out"=w514:errorcluster, "Acquisition out"=w546:refnum<class "Acquisition.lvclass">)  [unwired: 7 in]
                      n184 = call-dynamic "Write Interface.vi"("error in (no error)"=w516, "Interface.lvclass"=w528, "Channel in"=w531) -> ("error out"=w529:errorcluster, "Channel out"=w530:refnum<class "Channel.lvclass">)  [unwired: 7 in]
                      n185 = call-dynamic "Write #PREV Images.vi"("error in (no error)"=w496, "#PREV FRAMES"=w501, "Interface in"=w499) -> ("error out"=w495:errorcluster, "Interface out"=w498:refnum<class "Interface.lvclass">)  [unwired: 7 in]
                      n186 = call-dynamic "Read # Images.vi"("error in (no error)"=w481, "Interface in"=w484) -> ("error out"=w480:errorcluster, "# Images"=w485:u32, "Interface out"=w483:refnum<class "Interface.lvclass">)  [unwired: 7 in]
                      n187 = call-dynamic "Write #PREV Images.vi"("error in (no error)"=w480, "#PREV FRAMES"=w485, "Interface in"=w483) -> ("error out"=w479:errorcluster, "Interface out"=w482:refnum<class "Interface.lvclass">)  [unwired: 7 in]
                      n188 = call-dynamic "Write Interface.vi"("error in (no error)"=w495, "Interface.lvclass"=w498, "Channel in"=w510) -> ("error out"=w508:errorcluster, "Channel out"=w509:refnum<class "Channel.lvclass">)  [unwired: 7 in]
                      n189 = call-dynamic "Write Channel.vi"("error in (no error)"=w529, "Channel.lvclass"=w530, "Acquisition in"=w532) -> ("error out"=w513:errorcluster, "Acquisition out"=w515:refnum<class "Acquisition.lvclass">)  [unwired: 7 in]
                      n190 = call-dynamic "Write Interface.vi"("error in (no error)"=w479, "Interface.lvclass"=w482, "Channel in"=w493) -> ("error out"=w491:errorcluster, "Channel out"=w492:refnum<class "Channel.lvclass">)  [unwired: 7 in]
                      n191 = call-dynamic "Write Channel.vi"("error in (no error)"=w508, "Channel.lvclass"=w509, "Acquisition in"=w511) -> ("error out"=w475:errorcluster, "Acquisition out"=w476:refnum<class "Acquisition.lvclass">)  [unwired: 7 in]
                      n192 = call-dynamic "Write Channel.vi"("error in (no error)"=w491, "Channel.lvclass"=w492, "Acquisition in"=w494) -> ("error out"=w474:errorcluster, "Acquisition out"=w477:refnum<class "Acquisition.lvclass">)  [unwired: 7 in]
                    }
                  }
                  n193 = Bundle By Name(cluster=w308, "prev sequencias"=w300, "prev ciclos"=w315, "AcquisitionA"=w317, "AcquisitionB"=w313, "AcquisitionC"=w303, "AcquisitionD"=w304, "Instrument.lvclass"=w316) -> (w307:refnum<class "S4GUI.lvclass">)
                  n194 = Merge Errors(w312, w311, w302, w301, w310) -> (w309:errorcluster)
                }
              }
            }
            frame "TEST" {
              w577 = u32 1 ("ciclos")
              n195 = Unbundle By Name(w604) -> ("AcquisitionA"=w645:refnum<class "Acquisition.lvclass">, "AcquisitionB"=w644:refnum<class "Acquisition.lvclass">, "AcquisitionC"=w643:refnum<class "Acquisition.lvclass">, "AcquisitionD"=w642:refnum<class "Acquisition.lvclass">, "Instrument.lvclass"=w641:refnum<class "Instrument.lvclass">)
              n196 = call-dynamic "Read Channel.vi"("error in (no error)"=w590, "Acquisition in"=w645) -> ("error out"=w579:errorcluster, "Channel.lvclass"=w640:refnum<class "Channel.lvclass">, "Acquisition out"=w631:refnum<class "Acquisition.lvclass">)  [unwired: 7 in]
              n197 = call-dynamic "Read Channel.vi"("error in (no error)"=w590, "Acquisition in"=w644) -> ("error out"=w625:errorcluster, "Channel.lvclass"=w638:refnum<class "Channel.lvclass">, "Acquisition out"=w619:refnum<class "Acquisition.lvclass">)  [unwired: 7 in]
              n198 = disable-structure shown="Enabled" {
                disable-tunnel: w641 -> [w667 w669]
                disable-tunnel: [w665 w669] -> w598
                disable-tunnel: w590 -> [w664 w668]
                disable-tunnel: [w663 w668] -> w585
                frame Enabled {
                  # "OptSetector.Seq=<POSICAO ATUAL> faz a lâmina ficar \nonde está  (vide S4GUI:HandleObservationSync.vi - \nObs_state=303)."
                  n199 = call "Read WPROT.vi"("error in (no error)"=w664, "Instrument in"=w667) -> ("error out"=w657:errorcluster, "Opt_Selector.lvclass"=w662:refnum<class "Opt_Selector.lvclass">, "Instrument out"=w666:refnum<class "Instrument.lvclass">)  [unwired: 7 in]
                  n200 = call "Read id_pos.vi"("error in (no error)"=w657, "Optics in"=w662) -> ("error out"=w656:errorcluster, "id_pos"=w660:u32, "Optics out"=w661:refnum<class "Opt_Selector.lvclass">)  [unwired: 7 in]
                  n201 = Decrement(x=w660) -> (x-1=w652:u32)
                  n202 = Greater?(x=w652, y=u32 65535) -> (0:w653:bool)
                  n203 = Select(t=u32 0, s=w653, f=w652) -> (s? t:f=w655:u32)
                  n204 = Scale By Power Of 2(n=w655, x=ext 1.0) -> (x*2^n=w658:ext)
                  n205 = To Unsigned Word Integer(number=w658) -> (unsigned 16bit integer=w646:u16)
                  n206 = call-dynamic "Write sequencia.vi"("error in (no error)"=w656, "sequencia"=w646, "Opt_Selector in"=w661) -> ("error out"=w649:errorcluster, "Opt_Selector out"=w650:refnum<class "Opt_Selector.lvclass">)  [unwired: 7 in]
                  n207 = call-dynamic "Write sequencia_ant.vi"("error in (no error)"=w649, "sequencia_ant"=w646, "Opt_Selector in"=w650) -> ("error out"=w648:errorcluster, "Opt_Selector out"=w647:refnum<class "Opt_Selector.lvclass">)  [unwired: 7 in]
                  n208 = call "Write WPROT.vi"("error in (no error)"=w648, "Opt_Selector.lvclass"=w647, "Instrument in"=w666) -> ("error out"=w663:errorcluster, "Instrument out"=w665:refnum<class "Instrument.lvclass">)  [unwired: 7 in]
                }
                frame Disabled {
                }
              }
              n209 = call-dynamic "Write ciclos.vi"("error in (no error)"=w579, "ciclos"=u32 1, "Channel in"=w640) -> ("error out"=w573:errorcluster, "Channel out"=w575:refnum<class "Channel.lvclass">)  [unwired: 7 in]
              n210 = call-dynamic "Read Channel.vi"("error in (no error)"=w590, "Acquisition in"=w643) -> ("error out"=w615:errorcluster, "Channel.lvclass"=w637:refnum<class "Channel.lvclass">, "Acquisition out"=w618:refnum<class "Acquisition.lvclass">)  [unwired: 7 in]
              n211 = call-dynamic "Write ciclos.vi"("error in (no error)"=w625, "ciclos"=u32 1, "Channel in"=w638) -> ("error out"=w565:errorcluster, "Channel out"=w567:refnum<class "Channel.lvclass">)  [unwired: 7 in]
              n212 = call-dynamic "Read Channel.vi"("error in (no error)"=w590, "Acquisition in"=w642) -> ("error out"=w608:errorcluster, "Channel.lvclass"=w633:refnum<class "Channel.lvclass">, "Acquisition out"=w611:refnum<class "Acquisition.lvclass">)  [unwired: 7 in]
              n213 = call-dynamic "Write sequencias.vi"("error in (no error)"=w573, "sequencias"=u32 1, "Channel in"=w575) -> ("error out"=w572:errorcluster, "Channel out"=w574:refnum<class "Channel.lvclass">)  [unwired: 7 in]
              n214 = call-dynamic "Write ciclos.vi"("error in (no error)"=w615, "ciclos"=u32 1, "Channel in"=w637) -> ("error out"=w561:errorcluster, "Channel out"=w563:refnum<class "Channel.lvclass">)  [unwired: 7 in]
              n215 = call-dynamic "Write sequencias.vi"("error in (no error)"=w565, "sequencias"=u32 1, "Channel in"=w567) -> ("error out"=w564:errorcluster, "Channel out"=w566:refnum<class "Channel.lvclass">)  [unwired: 7 in]
              n216 = call-dynamic "Read Interface.vi"("error in (no error)"=w572, "Channel in"=w574) -> ("error out"=w628:errorcluster, "Interface.lvclass"=w634:refnum<class "Interface.lvclass">, "Channel out"=w630:refnum<class "Channel.lvclass">)  [unwired: 7 in]
              n217 = call-dynamic "Read Interface.vi"("error in (no error)"=w564, "Channel in"=w566) -> ("error out"=w624:errorcluster, "Interface.lvclass"=w635:refnum<class "Interface.lvclass">, "Channel out"=w621:refnum<class "Channel.lvclass">)  [unwired: 7 in]
              n218 = call-dynamic "Write sequencias.vi"("error in (no error)"=w561, "sequencias"=u32 1, "Channel in"=w563) -> ("error out"=w560:errorcluster, "Channel out"=w562:refnum<class "Channel.lvclass">)  [unwired: 7 in]
              n219 = call-dynamic "Write ciclos.vi"("error in (no error)"=w608, "ciclos"=u32 1, "Channel in"=w633) -> ("error out"=w557:errorcluster, "Channel out"=w559:refnum<class "Channel.lvclass">)  [unwired: 7 in]
              n220 = call-dynamic "Write # Images.vi"("error in (no error)"=w628, "# Images"=u32 1, "Interface in"=w634) -> ("error out"=w627:errorcluster, "Interface out"=w582:refnum<class "Interface.lvclass">)  [unwired: 7 in]
              n221 = call-dynamic "Read Interface.vi"("error in (no error)"=w560, "Channel in"=w562) -> ("error out"=w614:errorcluster, "Interface.lvclass"=w636:refnum<class "Interface.lvclass">, "Channel out"=w617:refnum<class "Channel.lvclass">)  [unwired: 7 in]
              n222 = call-dynamic "Write # Images.vi"("error in (no error)"=w624, "# Images"=u32 1, "Interface in"=w635) -> ("error out"=w623:errorcluster, "Interface out"=w583:refnum<class "Interface.lvclass">)  [unwired: 7 in]
              n223 = call-dynamic "Write sequencias.vi"("error in (no error)"=w557, "sequencias"=u32 1, "Channel in"=w559) -> ("error out"=w556:errorcluster, "Channel out"=w558:refnum<class "Channel.lvclass">)  [unwired: 7 in]
              n224 = call-dynamic "Write Interface.vi"("error in (no error)"=w627, "Interface.lvclass"=w582, "Channel in"=w630) -> ("error out"=w626:errorcluster, "Channel out"=w629:refnum<class "Channel.lvclass">)  [unwired: 7 in]
              n225 = call-dynamic "Write Interface.vi"("error in (no error)"=w623, "Interface.lvclass"=w583, "Channel in"=w621) -> ("error out"=w622:errorcluster, "Channel out"=w620:refnum<class "Channel.lvclass">)  [unwired: 7 in]
              n226 = call-dynamic "Write # Images.vi"("error in (no error)"=w614, "# Images"=u32 1, "Interface in"=w636) -> ("error out"=w613:errorcluster, "Interface out"=w581:refnum<class "Interface.lvclass">)  [unwired: 7 in]
              n227 = call-dynamic "Read Interface.vi"("error in (no error)"=w556, "Channel in"=w558) -> ("error out"=w607:errorcluster, "Interface.lvclass"=w632:refnum<class "Interface.lvclass">, "Channel out"=w610:refnum<class "Channel.lvclass">)  [unwired: 7 in]
              n228 = call-dynamic "Write Channel.vi"("error in (no error)"=w626, "Channel.lvclass"=w629, "Acquisition in"=w631) -> ("error out"=w589:errorcluster, "Acquisition out"=w602:refnum<class "Acquisition.lvclass">)  [unwired: 7 in]
              n229 = call-dynamic "Write Channel.vi"("error in (no error)"=w622, "Channel.lvclass"=w620, "Acquisition in"=w619) -> ("error out"=w588:errorcluster, "Acquisition out"=w601:refnum<class "Acquisition.lvclass">)  [unwired: 7 in]
              n230 = call-dynamic "Write Interface.vi"("error in (no error)"=w613, "Interface.lvclass"=w581, "Channel in"=w617) -> ("error out"=w612:errorcluster, "Channel out"=w616:refnum<class "Channel.lvclass">)  [unwired: 7 in]
              n231 = call-dynamic "Write # Images.vi"("error in (no error)"=w607, "# Images"=u32 1, "Interface in"=w632) -> ("error out"=w606:errorcluster, "Interface out"=w580:refnum<class "Interface.lvclass">)  [unwired: 7 in]
              n232 = call-dynamic "Write Channel.vi"("error in (no error)"=w612, "Channel.lvclass"=w616, "Acquisition in"=w618) -> ("error out"=w587:errorcluster, "Acquisition out"=w600:refnum<class "Acquisition.lvclass">)  [unwired: 7 in]
              n233 = call-dynamic "Write Interface.vi"("error in (no error)"=w606, "Interface.lvclass"=w580, "Channel in"=w610) -> ("error out"=w605:errorcluster, "Channel out"=w609:refnum<class "Channel.lvclass">)  [unwired: 7 in]
              n234 = call-dynamic "Write Channel.vi"("error in (no error)"=w605, "Channel.lvclass"=w609, "Acquisition in"=w611) -> ("error out"=w586:errorcluster, "Acquisition out"=w599:refnum<class "Acquisition.lvclass">)  [unwired: 7 in]
              n235 = Merge Errors(w589, w588, w587, w586, w585) -> (w584:errorcluster)
              n236 = Bundle By Name(cluster=w604, "RestauraTEST"=TRUE, "sequencias"=u32 1, "TotalCiclos"=w577, "ciclos"=w577, "AcquisitionA"=w602, "AcquisitionB"=w601, "AcquisitionC"=w600, "AcquisitionD"=w599, "Instrument.lvclass"=w598) -> (w603:refnum<class "S4GUI.lvclass">)
            }
            frame "FOCUS" {
              w691 = u32 1 ("ciclos")
              n237 = Unbundle By Name(w710) -> ("AcquisitionA"=w727:refnum<class "Acquisition.lvclass">, "AcquisitionB"=w726:refnum<class "Acquisition.lvclass">, "AcquisitionC"=w725:refnum<class "Acquisition.lvclass">, "AcquisitionD"=w724:refnum<class "Acquisition.lvclass">, "Instrument.lvclass"=w723:refnum<class "Instrument.lvclass">)
              n238 = call-dynamic "Read Channel.vi"("error in (no error)"=w700, "Acquisition in"=w727) -> ("error out"=w693:errorcluster, "Channel.lvclass"=w722:refnum<class "Channel.lvclass">, "Acquisition out"=w717:refnum<class "Acquisition.lvclass">)  [unwired: 7 in]
              n239 = call-dynamic "Read Channel.vi"("error in (no error)"=w700, "Acquisition in"=w726) -> ("error out"=w716:errorcluster, "Channel.lvclass"=w720:refnum<class "Channel.lvclass">, "Acquisition out"=w715:refnum<class "Acquisition.lvclass">)  [unwired: 7 in]
              n240 = call-dynamic "Write ciclos.vi"("error in (no error)"=w693, "ciclos"=u32 1, "Channel in"=w722) -> ("error out"=w688:errorcluster, "Channel out"=w689:refnum<class "Channel.lvclass">)  [unwired: 7 in]
              n241 = call-dynamic "Read Channel.vi"("error in (no error)"=w700, "Acquisition in"=w725) -> ("error out"=w713:errorcluster, "Channel.lvclass"=w719:refnum<class "Channel.lvclass">, "Acquisition out"=w714:refnum<class "Acquisition.lvclass">)  [unwired: 7 in]
              n242 = call-dynamic "Write ciclos.vi"("error in (no error)"=w716, "ciclos"=u32 1, "Channel in"=w720) -> ("error out"=w682:errorcluster, "Channel out"=w683:refnum<class "Channel.lvclass">)  [unwired: 7 in]
              n243 = call-dynamic "Read Channel.vi"("error in (no error)"=w700, "Acquisition in"=w724) -> ("error out"=w711:errorcluster, "Channel.lvclass"=w718:refnum<class "Channel.lvclass">, "Acquisition out"=w712:refnum<class "Acquisition.lvclass">)  [unwired: 7 in]
              n244 = call-dynamic "Write sequencias.vi"("error in (no error)"=w688, "sequencias"=u32 1, "Channel in"=w689) -> ("error out"=w676:errorcluster, "Channel out"=w677:refnum<class "Channel.lvclass">)  [unwired: 7 in]
              n245 = disable-structure shown="Enabled" {
                disable-tunnel: w723 -> [w740 w742]
                disable-tunnel: [w737 w742] -> w704
                disable-tunnel: w700 -> [w734 w741]
                disable-tunnel: [w733 w741] -> w695
                frame Disabled {
                  n246 = call "Read WPROT.vi"("error in (no error)"=w734, "Instrument in"=w740) -> ("error out"=w736:errorcluster, "Opt_Selector.lvclass"=w739:refnum<class "Opt_Selector.lvclass">, "Instrument out"=w738:refnum<class "Instrument.lvclass">)  [unwired: 7 in]
                  n247 = call-dynamic "Write sequencia.vi"("error in (no error)"=w736, "sequencia"=u16 0, "Opt_Selector in"=w739) -> ("error out"=w731:errorcluster, "Opt_Selector out"=w732:refnum<class "Opt_Selector.lvclass">)  [unwired: 7 in]
                  n248 = call-dynamic "Write sequencia_ant.vi"("error in (no error)"=w731, "sequencia_ant"=u16 0, "Opt_Selector in"=w732) -> ("error out"=w728:errorcluster, "Opt_Selector out"=w729:refnum<class "Opt_Selector.lvclass">)  [unwired: 7 in]
                  n249 = call "Write WPROT.vi"("error in (no error)"=w728, "Opt_Selector.lvclass"=w729, "Instrument in"=w738) -> ("error out"=w733:errorcluster, "Instrument out"=w737:refnum<class "Instrument.lvclass">)  [unwired: 7 in]
                }
                frame Enabled {
                  # "O START para a aba FOCUS é realizado no estado\nObs_state=360 em S4GUI:HandleObservationSync.vi e\nnão usa o valor de OptSelector.Seq (a lâmina fica onde está)."
                }
              }
              n250 = call-dynamic "Write ciclos.vi"("error in (no error)"=w713, "ciclos"=u32 1, "Channel in"=w719) -> ("error out"=w680:errorcluster, "Channel out"=w681:refnum<class "Channel.lvclass">)  [unwired: 7 in]
              n251 = call-dynamic "Write sequencias.vi"("error in (no error)"=w682, "sequencias"=u32 1, "Channel in"=w683) -> ("error out"=w674:errorcluster, "Channel out"=w675:refnum<class "Channel.lvclass">)  [unwired: 7 in]
              n252 = call-dynamic "Write sequencias.vi"("error in (no error)"=w680, "sequencias"=u32 1, "Channel in"=w681) -> ("error out"=w672:errorcluster, "Channel out"=w673:refnum<class "Channel.lvclass">)  [unwired: 7 in]
              n253 = call-dynamic "Write ciclos.vi"("error in (no error)"=w711, "ciclos"=u32 1, "Channel in"=w718) -> ("error out"=w678:errorcluster, "Channel out"=w679:refnum<class "Channel.lvclass">)  [unwired: 7 in]
              n254 = call-dynamic "Write sequencias.vi"("error in (no error)"=w678, "sequencias"=u32 1, "Channel in"=w679) -> ("error out"=w670:errorcluster, "Channel out"=w671:refnum<class "Channel.lvclass">)  [unwired: 7 in]
              n255 = call-dynamic "Write Channel.vi"("error in (no error)"=w676, "Channel.lvclass"=w677, "Acquisition in"=w717) -> ("error out"=w699:errorcluster, "Acquisition out"=w708:refnum<class "Acquisition.lvclass">)  [unwired: 7 in]
              n256 = call-dynamic "Write Channel.vi"("error in (no error)"=w674, "Channel.lvclass"=w675, "Acquisition in"=w715) -> ("error out"=w698:errorcluster, "Acquisition out"=w707:refnum<class "Acquisition.lvclass">)  [unwired: 7 in]
              n257 = call-dynamic "Write Channel.vi"("error in (no error)"=w672, "Channel.lvclass"=w673, "Acquisition in"=w714) -> ("error out"=w697:errorcluster, "Acquisition out"=w706:refnum<class "Acquisition.lvclass">)  [unwired: 7 in]
              n258 = call-dynamic "Write Channel.vi"("error in (no error)"=w670, "Channel.lvclass"=w671, "Acquisition in"=w712) -> ("error out"=w696:errorcluster, "Acquisition out"=w705:refnum<class "Acquisition.lvclass">)  [unwired: 7 in]
              n259 = Merge Errors(w699, w698, w697, w696, w695) -> (w694:errorcluster)
              n260 = Bundle By Name(cluster=w710, "RestauraTEST"=TRUE, "sequencias"=u32 1, "TotalCiclos"=w691, "ciclos"=w691, "AcquisitionA"=w708, "AcquisitionB"=w707, "AcquisitionC"=w706, "AcquisitionD"=w705, "Instrument.lvclass"=w704) -> (w709:refnum<class "S4GUI.lvclass">)
            }
          }
        }
        frame Default {
        }
      }
    }
    frame Error {
    }
  }
  "error out" <- w3
  "S4GUI out" <- w1
